vi "Build Preview.vi"(7 "Ambient":dbl, 8 "error in (no error)":errorcluster, 9 "Start Temp":dbl, 10 "Start Time":dbl, 11 "Rate Step in":refnum<class "Rate Duration.lvclass">) -> (0 "error out":errorcluster, 1 "End Temp":dbl, 2 "End Time":dbl, 3 "Rate Step out":refnum<class "Rate Duration.lvclass">, 4 "Step Plot Data":cluster{"Time":dbl[], "Value":dbl[]})   [LabVIEW 2018, in "Temp Recipe.lvlib" / "Rate Duration.lvclass"]
uses:
  Rate Duration.lvclass
  Rate Duration.lvclass/Rate Duration.ctl
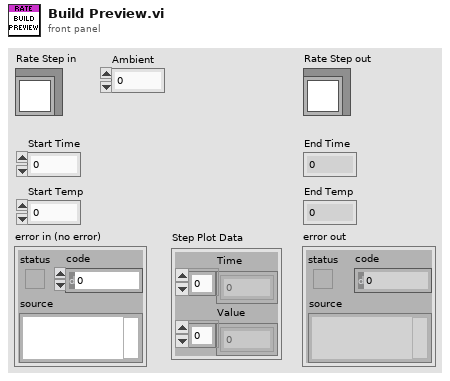
[diagram p1: front panel]
types:
  T1 = typedef "Temp Recipe.lvlib/Rate Duration.lvclass/Ref Data.ctl" = cluster{"Target":dbl, "Duration":dbl}
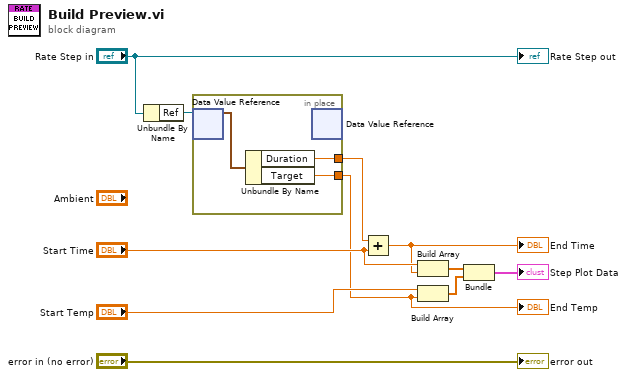
[diagram p0: block diagram]
diagram:
  n1 = Unbundle By Name("Rate Step in") -> ("Ref"=w10:refnum<data-value>)
  n2 = in-place {
    in-place-border: [w13] -> w8
    in-place-border: [w12] -> w1
    n3 = in-place-dvr #1(w10) -> (w14:T1)  [unwired: 1 out]
    n4 = Unbundle By Name(w14) -> ("Duration"=w13:dbl, "Target"=w12:dbl)
    n5 = in-place-dvr #1() -> ()  [unwired: 1 in, 2 out]
  }
  "End Temp" <- w1
  n6 = Add(x=w8, y="Start Time") -> (x+y=w6:dbl)
  "End Time" <- w6
  n7 = Build Array("Start Time", w6) -> (w4:dbl[])
  n8 = Build Array("Start Temp", w1) -> (w3:dbl[])
  n9 = Bundle(w4, w3) -> (→"Step Plot Data":cluster{dbl[], dbl[]})  [unwired: 1 in]
  "error out" <- "error in (no error)"
  "Rate Step out" <- "Rate Step in"
